vi "Get Enclave.vi"(11 "Lossless in":refnum<class "Lossless.lvclass">) -> (2 "Enclave":refnum<class "Enclave.lvclass">)   [LabVIEW 2022 SP3, in "Enclave.lvlib" / "Lossless.lvclass"]
uses:
  Lossless.lvclass
  Enclave/Enclave.lvclass
  Lossless.lvclass/Lossless.ctl
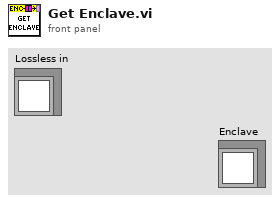
[diagram p1: front panel]
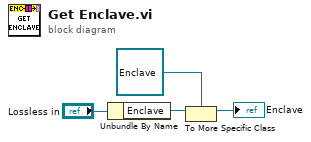
[diagram p0: block diagram]
diagram:
  n1 = Unbundle By Name("Lossless in") -> ("Enclave"=w3:refnum<class>)
  n2 = To More Specific Class(target class=refnum<class "Enclave.lvclass"> refnum ("Enclave.lvlib:Enclave.lvclass"), reference=w3) -> (specific class reference=→"Enclave":refnum<class "Enclave.lvclass">)  [unwired: 1 in, 1 out]
